vi "test Get Error Text.vi"(11 "Test Case In":refnum<class "Test PCANBasic.lvclass">) -> (0 "error out":errorcluster, 3 "Test Case Out":refnum<class "Test PCANBasic.lvclass">)   [LabVIEW 2020, in "Test PCANBasic.lvclass"]
uses:
  Test PCANBasic.lvclass
  C:/Program Files/National Instruments/LabVIEW 2026/vi.lib/Astemes/LUnit/Test Case.lvclass
  <vilib>/Astemes/LUnit/Test Case.lvclass/Test Case.ctl
  Global PCAN Channel.vi
  source/PCANBasic.lvlib
  <vilib>/Astemes/LUnit/Test Case.lvclass
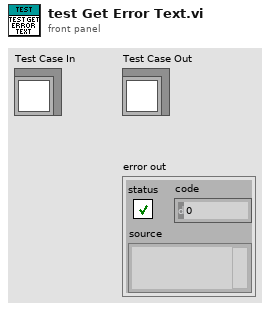
[diagram p1: front panel]
types:
  T1 = typedef "PCANBasic.lvlib/TPCANHandle.ctl" = u16
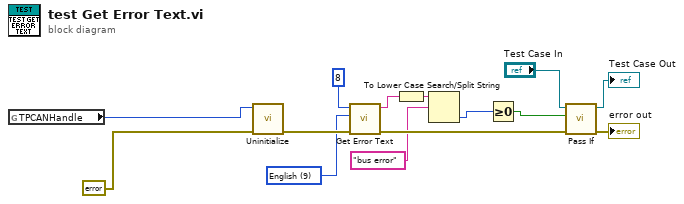
[diagram p0: block diagram]
diagram:
  w7 = u16 9 items=["Neutral"=0, "German"=7, "English"=9, "Spanish"=16, "French"=18, "Italian"=22] ("Language")
  n1 = global read "Global PCAN Channel.vi" "TPCANHandle"() -> (w10:T1)
  n2 = call "Uninitialize.vi"("error in"=errorcluster {"status"=FALSE, "code"=0, "source"=""}, "TPCANHandle in"=w10) -> ("error out"=w9:errorcluster)  [unwired: 8 in, 1 out]
  n3 = call "Get Error Text.vi"("error in"=w9, "Language"=w7, "PCAN Error Code"=u32 8) -> ("error out"=w8:errorcluster, "PCAN Error Text"=w5:string)  [unwired: 7 in]
  n4 = To Lower Case(string=w5) -> (all lower case string=w1:string)
  n5 = Search/Split String(string=w1, search string/char (-)="bus error") -> (offset of match=w3:i32)  [unwired: 1 in, 2 out]
  n6 = Greater Or Equal To 0?(x=w3) -> (x >= 0?=w2:bool)
  n7 = call <vilib>:"Pass If.vi"("error in (no error)"=w8, "Pass?"=w2, "LUnit Test Case In"="Test Case In") -> ("error out"=→"error out":errorcluster, "LUnit Test Case Out"=→"Test Case Out":refnum<class "Test PCANBasic.lvclass">)  [unwired: 7 in]
